vi "WRITE_LOG_FILE.vi"(0 "file path (use dialog)":path, 1 "OPERADOR":string, 4 "Resultado test":bool, 5 "ASIC QR CODE":string, 7 "HORA COMIENZO":timestamp, 9 "error in":errorcluster) -> (19 "error out":errorcluster)   [LabVIEW 2019]
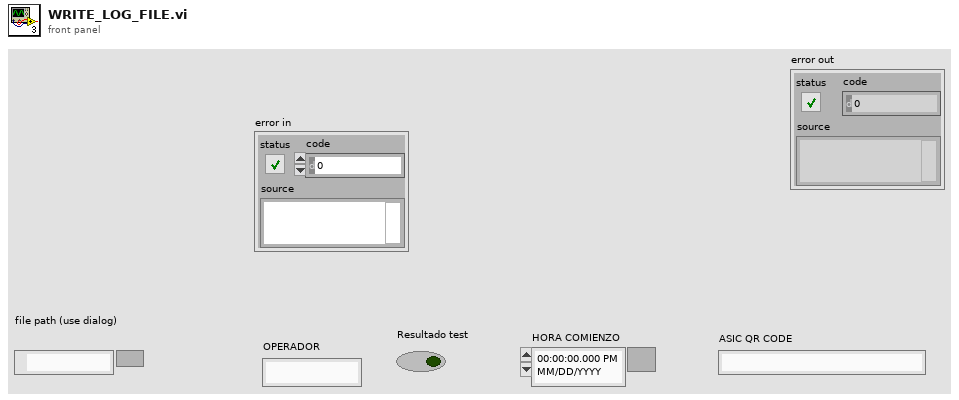
[diagram p1: front panel]
types:
  T1 = enum16{"open", "replace", "create", "open or create", "replace or create", "replace or create with confirmation"}
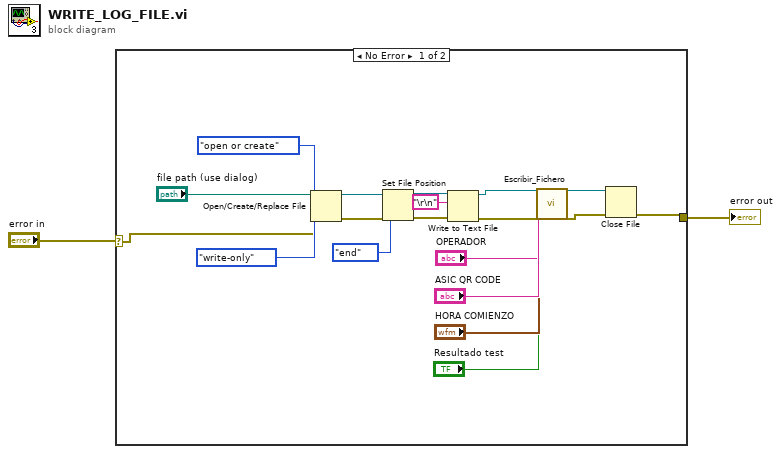
[diagram p0: block diagram]
diagram:
  n1 = case shown="No Error" "error in" {
    selector: "error in" -> [w6 w22]
    tunnel: [w3 w22] -> w2
    frame No Error {
      n2 = Open/Create/Replace File(file path (use dialog)="file path (use dialog)", error in=w6, operation (0:open)=T1."open or create", access (0:read/write)=enum16{"read/write", "read-only", "write-only"}."write-only") -> (refnum out=w17:refnum<file>, error out=w18:errorcluster)  [unwired: 2 in, 1 out]
      n3 = Set File Position(refnum=w17, from (0:start)=enum16{"start", "end", "current"}."end", error in=w18) -> (refnum out=w14:refnum<file>, error out=w15:errorcluster)  [unwired: 1 in]
      n4 = Write to Text File(file (use dialog)=w14, text="\r\n", error in=w15) -> (refnum out=w13:refnum<file>, error out=w8:errorcluster)  [unwired: 1 in, 1 out]
      n5 = call "Escribir_Fichero.vi"("refnum FILE"=w13, "ASIC QR CODE"="ASIC QR CODE", "HORA COMIENZO"="HORA COMIENZO", "OPERADOR"="OPERADOR", "Resultado test"="Resultado test", "error in (no error)"=w8) -> ("refnum out"=w5:refnum<file>, "error out"=w4:errorcluster)  [unwired: 20 in]
      n6 = Close File(refnum=w5, error in=w4) -> (error out=w3:errorcluster)  [unwired: 1 out]
    }
    frame Error {
    }
  }
  "error out" <- w2
